vi "Calculate UV In Pixels.vi"(7 "Texture Dimensions":T2, 11 "UV":T3 {"v" min=0 max=1 step=0.1; "u" min=0 max=1 step=0.1}) -> (3 "Pixels":T1)   [LabVIEW 2020, in "Raster (FPGA).lvlib"]
uses:
  Raster (FPGA).lvlib
  UV.ctl
  Rectangle Dimensions.ctl
  Point 2D (SGL).ctl
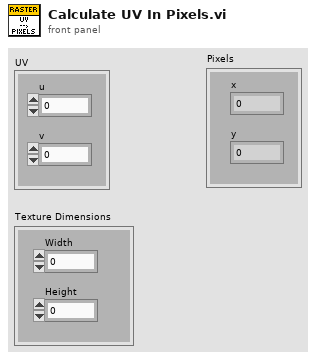
[diagram p1: front panel]
types:
  T1 = typedef "Raster (FPGA).lvlib/Point 2D (SGL).ctl" = cluster{"x":sgl, "y":sgl}
  T2 = typedef "Raster (FPGA).lvlib/Rectangle Dimensions.ctl" = cluster{"Width":u32, "Height":u32}
  T3 = typedef "Raster (FPGA).lvlib/UV.ctl" = cluster{"u":sgl, "v":sgl}
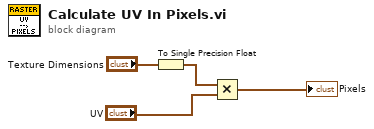
[diagram p0: block diagram]
diagram:
  n1 = To Single Precision Float(number="Texture Dimensions") -> (single precision float=w3:cluster{"Width":sgl, "Height":sgl})
  n2 = Multiply(x=w3, y="UV") -> (x*y=→"Pixels":T3)
